vi "Set TCP Messaging Info.vi"(8 "error in (no error)":errorcluster, 10 "TCP Messaging Info":T1, 11 "Node Config in":refnum<class "Node Config.lvclass">) -> (0 "error out":errorcluster, 3 "Node Config out":refnum<class "Node Config.lvclass">)   [LabVIEW 2020, in "Vecto.lvlib" / "Node Config.lvclass"]
uses:
  Node Config.lvclass
  Node Config.lvclass/Node Config.ctl
  TCP Messaging Info.ctl
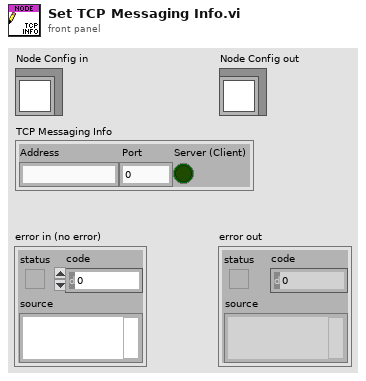
[diagram p1: front panel]
types:
  T1 = typedef "Vecto.lvlib/Node Config.lvclass/TCP Messaging Info.ctl" = cluster{"Address":string, "Port":u16, "Server (Client)":bool}
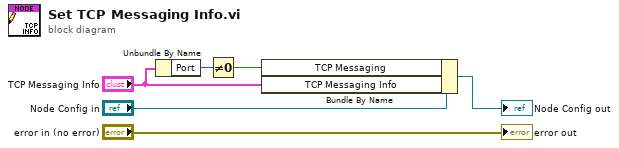
[diagram p0: block diagram]
diagram:
  n1 = Unbundle By Name("TCP Messaging Info") -> ("Port"=w1:u16)
  n2 = Not Equal To 0?(x=w1) -> (x != 0?=w2:bool)
  n3 = Bundle By Name(cluster="Node Config in", "TCP Messaging"=w2, "TCP Messaging Info"="TCP Messaging Info") -> (→"Node Config out":refnum<class "Node Config.lvclass">)
  "error out" <- "error in (no error)"
